vi "MultiPAS-III.vi"() -> ()   [LabVIEW 2011]
uses:
  <vilib>/Analysis/4window.llb/windowTd.ctl
  sub/QMH/QMH Add Message to Queue (Single Element).vi
  sub/QMH/QMH Add Message to Queue (Array).vi
  <vilib>/measure/maspectr.llb/FFT Spectrum (Mag-Phase) for 1 Chan.vi
  sub/fftGetMags.vi
  sub/rollingAverage_III.vi
  sub/micUnbundle_III.vi
  <vilib>/Instr/_visa.llb/VISA Configure Serial Port (Instr).vi
  sub/absCalcPlot_III.vi
  sub/pdNormalize_III.vi
  <vilib>/measure/NI_MAPro.lvlib
  <vilib>/Analysis/NI_AALPro.lvlib
panel:
  out "PAS Save":bool caption="Overtemp"
  in  "Data 2":i32[][](array[numeric])=[[-16374, -7248, 2543, 12030, 20279, 26487, 30037, 30583, 28073, 22744, 15131, 5976, -3818, -13288, -21504, -27663, -31155, -31636, -29064, -23686, -16036, -6862, 2936, 12388, 20571, 26684, 30122, 30546, 27911, 22483, 14793, 5595, -4207, -13644, -21795, -27855, -31232, -31591, -28898, -23423, -15695, -6476, 3323, 12743, 20858, 26873, 30194, 30492, 27744, 22213, 14447, 5207, -4597, -14002, -22082, -28044, -31304, -31540, -28731, -23149, -15348, -6093, 3713, 13101, 21145, 27063, 30265, 30442, 27576, 21943, 14103, 4822, -4984, -14354, -22365, -28230, -31373, -31485, -28556, -22876, -14998, -5702, 4104, 13452, 21428, 27245, 30335, 30388, 27400, 21669, 13754, 4435, -5375, -14705, -22643, -28407, -31436, -31426, -28378, -22598, -14648, -5314, 4497, 13803, 21706, 27423, 30394, 30325, 27221, 21390, 13402, 4045, -5763, -15056, -22921, -28586, -31496, -31361, -28198, -22319, -14297, -4924, 4879, 14151, 21982, 27597, 30451, 30257, 27038, 21107, 13050, 3658, -6149, -15402, -23193, -28754, -31546, -31290, -28010, -22033, -13944, -4536, 5266, 14498, 22252, 27767, 30500, 30184, 26849, 20821, 12696, 3267, -6535, -15748, -23462, -28924, -31596, -31216, -27821, -21748, -13587, -4147, 5653, 14838, 22519, 27930, 30549, 30110, 26658, 20535, 12337, 2878, -6919, -16089, -23727, -29087, -31641, -31137, -27627, -21457, -13229, -3753, 6038, 15181, 22786, 28093, 30591, 30031, 26461, 20243, 11979, 2485, -7303, -16428, -23991, -29244, -31678, -31053, -27426, -21159, -12867, -3360, 6424, 15524, 23043, 28252, 30633, 29946, 26262, 19946, 11617, 2096, -7686, -16764, -24246, -29398, -31712, -30964, -27224, -20862, -12503, -2971, 6803, 15859, 23301, 28401, 30661, 29852, 26058, 19648, 11254, 1703, -8069, -17099, -24500, -29547, -31741, -30870, -27018, -20562, -12138, -2575, 7188, 16192, 23556, 28549, 30689, 29756, 25848, 19348, 10891, 1312, -8448, -17430, -24753, -29691, -31765, -30773, -26806, -20259, -11775, -2186, 7566, 16521, 23801, 28690, 30709, 29656, 25634, 19038, 10523, 919, -8831, -17762, -24997, -29833, -31788, -30672, -26593, -19955, -11409, -1792, 7944, 16850, 24047, 28830, 30724, 29548, 25416, 18729, 10152, 523, -9212, -18092, -25245, -29969, -31805, -30566, -26375, -19647, -11041, -1403, 8319, 17173, 24287, 28963, 30734, 29436, 25192, 18418, 9781, 130, -9587, -18413, -25481, -30101, -31814, -30449, -26150, -19332, -10666, -1007, 8697, 17497, 24524, 29090, 30745, 29325, 24968, 18105, 9408, -263, -9962, -18735, -25718, -30228, -31820, -30334, -25921, -19016, -10296, -618, 9072, 17814, 24756, 29213, 30746, 29202, 24738, 17787, 9036, -657, -10338, -19058, -25951, -30350, -31818, -30214, -25690, -18699, -9922, -224, 9442, 18128, 24984, 29330, 30738, 29078, 24502, 17466, 8658, -1050, -10710, -19371, -26178, -30467, -31814, -30088, -25458, -18382, -9550, 167, 9812, 18440, 25206, 29443, 30732, 28947, 24264, 17143, 8281, -1445, -11083, -19685, -26404, -30581, -31807, -29959, -25221, -18059, -9175, 556, 10178, 18750, 25426, 29548, 30718, 28809, 24018, 16812, 7901, -1842, -11457, -19996, -26624, -30690, -31795, -29824, -24980, -17733, -8799, 950, 10549, 19058, 25643, 29655, 30700, 28673, 23773, 16484, 7523, -2235, -11824, -20304, -26840, -30793, -31772, -29682, -24731, -17402, -8415, 1341, 10916, 19363, 25856, 29755, 30677, 28528, 23522, 16151, 7141, -2626, -12191, -20607, -27051, -30891, -31746, -29536, -24481, -17070, -8035, 1733, 11280, 19664, 26064, 29851, 30648, 28381, 23272, 15818, 6762, -3019, -12555, -20906, -27258, -30984, -31717, -29391, -24226, -16736, -7655, 2128, 11641, 19962, 26270, 29940, 30615, 28229, 23013, 15483, 6376, -3409, -12914, -21204, -27459, -31071, -31684, -29236, -23967, -16398, -7271, 2515, 12005, 20258, 26468, 30024, 30577, 28072, 22753, 15143, 5990, -3802, -13276, -21497, -27660, -31157, -31643, -29076, -23707, -16058, -6886, 2908, 12363, 20550, 26666, 30107, 30536, 27914, 22489, 14805, 5607, -4192, -13633, -21787, -27849, -31230, -31597, -28911, -23438, -15716, -6501, 3298, 12719, 20839, 26858, 30182, 30488, 27744, 22223, 14459, 5225, -4579, -13988, -22071, -28040, -31304, -31549, -28743, -23167, -15368, -6113, 3693, 13076, 21126, 27047, 30255, 30438, 27576, 21950, 14113, 4837, -4971, -14340, -22354, -28224, -31375, -31494, -28570, -22895, -15022, -5725, 4080, 13430, 21408, 27230, 30324, 30384, 27402, 21676, 13766, 4449, -5360, -14694, -22636, -28409, -31440, -31436, -28397, -22617, -14674, -5338, 4467, 13781, 21686, 27408, 30385, 30320, 27224, 21398, 13418, 4062, -5748, -15044, -22913, -28584, -31498, -31368, -28212, -22339, -14321, -4948, 4856, 14131, 21963, 27583, 30440, 30254, 27042, 21118, 13062, 3669, -6137, -15390, -23183, -28751, -31551, -31297, -28024, -22049, -13962, -4556, 5245, 14476, 22235, 27754, 30497, 30186, 26857, 20834, 12710, 3283, -6519, -15733, -23453, -28921, -31600, -31226, -27837, -21765, -13610, -4168, 5628, 14820, 22502, 27918, 30540, 30109, 26664, 20544, 12354, 2891, -6906, -16074, -23719, -29085, -31646, -31148, -27642, -21475, -13251, -3777, 6014, 15160, 22765, 28078, 30583, 30027, 26468, 20251, 11994, 2501, -7292, -16415, -23980, -29242, -31682, -31064, -27443, -21181, -12892, -3386, 6397, 15501, 23026, 28238, 30624, 29944, 26269, 19959, 11633, 2110, -7673, -16753, -24239, -29395, -31719, -30974, -27239, -20882, -12528, -2993, 6782, 15835, 23285, 28390, 30651, 29852, 26063, 19660, 11271, 1720, -8053, -17087, -24493, -29546, -31746, -30880, -27031, -20583, -12163, -2599, 7166, 16173, 23538, 28538, 30684, 29758, 25853, 19356, 10906, 1327, -8433, -17416, -24743, -29688, -31769, -30782, -26821, -20280, -11797, -2208, 7543, 16501, 23786, 28680, 30704, 29656, 25642, 19053, 10540, 936, -8814, -17747, -24989, -29827, -31787, -30678, -26606, -19973, -11430, -1817, 7923, 16829, 24031, 28819, 30721, 29552, 25424, 18746, 10174, 543, -9191, -18072, -25231, -29962, -31802, -30567, -26384, -19660, -11057, -1422, 8302, 17159, 24274, 28952, 30738, 29443, 25205, 18435, 9801, 150, -9568, -18401, -25472, -30095, -31811, -30457, -26163, -19349, -10687, -1031, 8679, 17481, 24511, 29082, 30742, 29327, 24979, 18121, 9431, -241, -9943, -18717, -25707, -30221, -31815, -30337, -25930, -19029, -10312, -631, 9058, 17802, 24745, 29207, 30746, 29209, 24750, 17805, 9057, -634, -10316, -19037, -25937, -30340, -31814, -30217, -25700, -18713, -9939, -240, 9429, 18117, 24976, 29328, 30740, 29088, 24519, 17486, 8682, -1027, -10688, -19352, -26164, -30458, -31810, -30091, -25465, -18390, -9561, 154, 9800, 18433, 25201, 29442, 30735, 28959, 24282, 17165, 8308, -1420, -11063, -19665, -26386, -30570, -31801, -29961, -25227, -18068, -9185, 547, 10171, 18745, 25424, 29552, 30726, 28825, 24038, 16835, 7925, -1815, -11429, -19974, -26608, -30681, -31789, -29826, -24984, -17741, -8807, 938, 10536, 19047, 25636, 29657, 30708, 28685, 23794, 16510, 7550, -2205, -11798, -20280, -26821, -30782, -31766, -29684, -24737, -17411, -8429, 1331, 10906, 19356, 25851, 29758, 30684, 28544, 23546, 16178, 7169, -2598, -12162, -20582, -27035, -30879, -31744, -29540, -24485, -17080, -8048, 1721, 11267, 19655, 26061, 29852, 30654, 28395, 23291, 15843, 6786, -2993, -12527, -20884, -27240, -30974, -31713, -29390, -24230, -16744, -7662, 2115, 11635, 19957, 26268, 29945, 30624, 28246, 23035, 15509, 6406, -3382, -12889, -21180, -27444, -31061, -31677, -29236, -23975, -16408, -7284], [-19329, -1252, 17344, 29341, 30145, 19451, 1353, -17227, -29174, -29920, -19175, -1056, 17506, 29408, 30095, 19300, 1159, -17387, -29238, -29860, -19019, -860, 17671, 29475, 30037, 19143, 960, -17553, -29307, -29809, -18866, -664, 17832, 29545, 29987, 18991, 771, -17707, -29365, -29749, -18707, -466, 17992, 29605, 29926, 18832, 570, -17873, -29434, -29694, -18556, -272, 18151, 29670, 29869, 18676, 375, -18031, -29495, -29633, -18395, -75, 18310, 29729, 29809, 18516, 175, -18194, -29561, -29579, -18238, 120, 18469, 29792, 29750, 18362, -17, -18347, -29617, -29515, -18076, 316, 18629, 29848, 29682, 18197, -218, -18510, -29679, -29456, -17921, 513, 18787, 29910, 29626, 18042, -408, -18664, -29734, -29388, -17757, 709, 18941, 29965, 29560, 17875, -609, -18823, -29791, -29326, -17600, 904, 19095, 30023, 29495, 17717, -802, -18975, -29845, -29260, -17434, 1099, 19251, 30075, 29425, 17551, -1001, -19131, -29901, -29194, -17277, 1296, 19408, 30130, 29359, 17393, -1193, -19284, -29953, -29124, -17112, 1491, 19560, 30184, 29290, 17225, -1392, -19440, -30008, -29056, -16949, 1686, 19713, 30237, 29226, 17069, -1581, -19587, -30054, -28982, -16781, 1883, 19866, 30287, 29151, 16898, -1781, -19742, -30107, -28913, -16616, 2079, 20018, 30337, 29082, 16737, -1973, -19888, -30152, -28838, -16449, 2275, 20167, 30383, 29006, 16564, -2174, -20041, -30200, -28765, -16282, 2471, 20321, 30430, 28934, 16403, -2364, -20187, -30243, -28688, -16113, 2669, 20465, 30470, 28853, 16230, -2568, -20341, -30294, -28618, -15953, 2860, 20615, 30519, 28783, 16070, -2755, -20486, -30335, -28537, -15779, 3057, 20760, 30560, 28700, 15892, -2956, -20637, -30378, -28461, -15613, 3252, 20909, 30605, 28628, 15730, -3145, -20777, -30418, -28377, -15440, 3446, 21054, 30645, 28543, 15557, -3345, -20927, -30460, -28299, -15271, 3643, 21199, 30686, 28465, 15391, -3534, -21066, -30495, -28215, -15100, 3839, 21345, 30722, 28380, 15214, -3734, -21213, -30534, -28134, -14928, 4032, 21487, 30760, 28300, 15044, -3926, -21355, -30570, -28052, -14757, 4225, 21627, 30792, 28209, 14870, -4123, -21501, -30607, -27968, -14586, 4419, 21768, 30832, 28129, 14702, -4314, -21637, -30639, -27880, -14413, 4612, 21907, 30859, 28040, 14521, -4515, -21780, -30675, -27796, -14241, 4804, 22048, 30895, 27953, 14352, -4702, -21919, -30705, -27707, -14064, 4999, 22187, 30922, 27859, 14172, -4900, -22060, -30739, -27620, -13892, 5193, 22326, 30954, 27773, 14003, -5090, -22194, -30765, -27524, -13712, 5386, 22462, 30981, 27679, 13823, -5285, -22333, -30794, -27436, -13538, 5580, 22600, 31013, 27591, 13650, -5476, -22466, -30820, -27343, -13363, 5770, 22732, 31033, 27491, 13468, -5673, -22605, -30848, -27251, -13187, 5964, 22870, 31060, 27401, 13292, -5863, -22736, -30870, -27155, -13010, 6156, 23000, 31079, 27299, 13111, -6058, -22873, -30895, -27060, -12833, 6347, 23134, 31104, 27208, 12936, -6248, -23004, -30918, -26965, -12652, 6536, 23260, 31120, 27106, 12753, -6444, -23136, -30939, -26865, -12472, 6729, 23395, 31148, 27011, 12578, -6634, -23266, -30959, -26766, -12296, 6919, 23523, 31161, 26907, 12392, -6830, -23402, -30982, -26665, -12115, 7109, 23652, 31180, 26809, 12213, -7016, -23524, -30992, -26564, -11932, 7301, 23777, 31195, 26704, 12032, -7210, -23655, -31011, -26464, -11755, 7492, 23907, 31211, 26605, 11855, -7395, -23778, -31024, -26358, -11573, 7680, 24031, 31218, 26494, 11665, -7592, -23908, -31039, -26258, -11392, 7871, 24158, 31237, 26394, 11491, -7775, -24031, -31050, -26153, -11210, 8063, 24281, 31247, 26285, 11302, -7972, -24159, -31062, -26046, -11027, 8250, 24407, 31258, 26180, 11124, -8157, -24276, -31067, -25937, -10841, 8438, 24526, 31265, 26071, 10936, -8347, -24401, -31078, -25829, -10659, 8630, 24649, 31275, 25965, 10755, -8533, -24522, -31087, -25721, -10474, 8816, 24770, 31280, 25853, 10566, -8726, -24641, -31091, -25608, -10290, 9003, 24891, 31287, 25746, 10386, -8910, -24756, -31095, -25498, -10105, 9192, 25008, 31287, 25627, 10196, -9102, -24881, -31101, -25386, -9919, 9381, 25127, 31296, 25521, 10019, -9284, -24994, -31099, -25268, -9732, 9570, 25243, 31293, 25403, 9826, -9476, -25113, -31105, -25157, -9544, 9756, 25359, 31298, 25291, 9645, -9655, -25225, -31099, -25040, -9359, 9942, 25473, 31291, 25167, 9453, -9847, -25341, -31102, -24926, -9173, 10124, 25586, 31294, 25057, 9269, -10029, -25450, -31095, -24809, -8986, 10310, 25696, 31284, 24931, 9078, -10218, -25564, -31094, -24688, -8798, 10497, 25812, 31287, 24819, 8896, -10399, -25673, -31085, -24567, -8608, 10682, 25922, 31278, 24698, 8703, -10587, -25785, -31080, -24448, -8422, 10866, 26033, 31274, 24582, 8522, -10765, -25890, -31067, -24321, -8230, 11050, 26140, 31263, 24455, 8325, -10952, -26001, -31064, -24201, -8040, 11234, 26248, 31255, 24338, 8142, -11132, -26106, -31054, -24079, -7852, 11417, 26353, 31243, 24207, 7948, -11316, -26217, -31041, -23952, -7662, 11601, 26464, 31236, 24089, 7763, -11494, -26315, -31025, -23829, -7471, 11782, 26562, 31217, 23957, 7567, -11682, -26422, -31014, -23702, -7282, 11962, 26667, 31205, 23834, 7383, -11859, -26521, -30998, -23575, -7092, 12144, 26770, 31187, 23704, 7186, -12043, -26626, -30981, -23444, -6900, 12328, 26875, 31176, 23582, 7003, -12218, -26724, -30962, -23316, -6709, 12505, 26971, 31154, 23446, 6805, -12401, -26825, -30946, -23189, -6517, 12687, 27073, 31139, 23322, 6620, -12576, -26919, -30922, -23054, -6323, 12867, 27170, 31114, 23185, 6422, -12760, -27022, -30904, -22923, -6132, 13047, 27272, 31096, 23060, 6237, -12934, -27114, -30879, -22790, -5940, 13222, 27362, 31068, 22921, 6041, -13116, -27212, -30855, -22657, -5748, 13401, 27461, 31048, 22790, 5853, -13289, -27302, -30828, -22522, -5555, 13577, 27549, 31019, 22652, 5652, -13472, -27398, -30806, -22388, -5362, 13753, 27645, 30995, 22521, 5463, -13642, -27487, -30776, -22248, -5169, 13928, 27733, 30963, 22376, 5266, -13823, -27584, -30750, -22113, -4975, 14106, 27828, 30937, 22246, 5082, -13992, -27669, -30717, -21974, -4782, 14280, 27914, 30902, 22101, 4880, -14174, -27760, -30689, -21837, -4588, 14454, 28006, 30875, 21965, 4692, -14340, -27843, -30653, -21693, -4391, 14631, 28092, 30840, 21822, 4494, -14519, -27934, -30620, -21552, -4198, 14805, 28179, 30808, 21688, 4308, -14687, -28015, -30582, -21410, -4004, 14975, 28262, 30770, 21540, 4106, -14861, -28103, -30548, -21268, -3808, 15149, 28349, 30739, 21402, 3916, -15032, -28183, -30512, -21124, -3614, 15319, 28430, 30697, 21255, 3715, -15205, -28267, -30475, -20982, -3421, 15490, 28513, 30664, 21116, 3524, -15376, -28348, -30435, -20837, -3225, 15660, 28592, 30617, 20962, 3327, -15550, -28432, -30397, -20695, -3032, 15829, 28673, 30581, 20820, 3134, -15711, -28506, -30353, -20546, -2837, 15994, 28746, 30530, 20669, 2933, -15887, -28585, -30311, -20400, -2641, 16167, 28828, 30496, 20528, 2745, -16052, -28660, -30264, -20248, -2445, 16335, 28901, 30445, 20376, 2544, -16221, -28737, -30219, -20102, -2250, 16505, 28983, 30406, 20231, 2357, -16381, -28808, -30171, -19950, -2053, 16670, 29053, 30355, 20075, 2154, -16552, -28883, -30127, -19803, -1859, 16835, 29128, 30308, 19930, 1965, -16714, -28952, -30073, -19650, -1663, 17001, 29192, 30255, 19772, 1764, -16881, -29028, -30026, -19496, -1467, 17165, 29268, 30208, 19626, 1572, -17043, -29095, -29977, -19346]]
  out "Filtering":bool caption="Time has Elapsed"
  in  "Switch Filter":bool
  in  "Auto Filter":bool
  out "Elapsed Time (min)":dbl caption="Elapsed Time (s)" format="%#.1g"
  in  "Filter Length (min)":dbl=6.0 caption="Time Target (s)"
  in  "Sample Length (min)":dbl=24.0 caption="Time Target (s)" format="%#.1f"
  out "Time has Elapsed":bool
  in  "Time Target (s)":dbl=1.0
  in  "sweep":bool
  in  "All Emit":bool
  in  "Alignment Mode":bool
  in  "782 Emission":bool
  in  "782 Power (mW)":dbl(slide)=100.0 min=0.0 max=100.0 step=1.0 scale=0.0..100.0
  in  "532 Emission":bool
  in  "532 Power (mW)":dbl(slide)=100.0 min=0.0 max=100.0 step=1.0 scale=0.0..100.0
  in  "423 Power (mW)":dbl(slide)=100.0 min=0.0 max=100.0 step=1.0 scale=0.0..100.0
  in  "423 Emission":bool
  out "Overtemp":bool
  in  "Tab Control":T1(tab)=enum."Frequency Sweep"
  out "Error Console":T2
  out "pd":path caption="Photodiode File Path"
  out "mic":path caption="Microphone File Path"
  out "processed":path caption="Processed Data File Path"
  out "sweeps":path caption="Frequency Sweeps File Path"
  out "Laser Temperatures":T3(graph)
  in  "pd id":u32=1
  in  "mic id":u32
  in  "mic cal, scu":dbl=5.41531278804282e-05 format="%#_3e"
  in  "mic cal, scu":dbl=5.59307241877627e-05 format="%#_3e"
  in  "423 Port":refnum<visa-resource-name>="COM86"
  in  "532 Port":refnum<visa-resource-name>="COM85"
  in  "782 Port":refnum<visa-resource-name>="COM84"
  in  "Teensy Port":refnum<visa-resource-name>="COM87"
  in  "Save Data":bool
  in  "405 PD Cal 3":dbl=0.237
  in  "532 PD Cal 3":dbl=0.454
  in  "660 PD Cal 3":dbl=0.793
  out "freqscan":cluster{i32[], "Best Gaussian Fit":dbl[]}[](graph) caption="Frequency Sweep"
  out "sweep progress":dbl(slide) scale=0.0..1.0
  in  "Autosweep?":bool=TRUE
  in  "set freqs":bool
  out "Calculated Resonance (Hz)":dbl=1370.0
  in  "Data Start Frequency (Hz)":i32=1355
  in  "Data End Frequency (Hz)":i32=1385
  in  "423 F (Hz)":i32=1368
  in  "532 F (Hz)":i32=1372
  in  "785 F (Hz)":i32=1370
  in  "Chart Rolling Average":i32=64
  out "pdwave":waveform(i32)(graph) caption="Photodiode Waveform"
  out "pd ts":cluster{dbl, dbl, dbl}(graph)
  out "pdfft":cluster{"f0":dbl, "df":dbl, "magnitude":dbl[]}(graph) caption="Photodiode FFT"
  in  "rollavg":i32=16 caption="Dispaly Averaging (Transfers to Absorption Data!)"
  out "mic ts":T4(graph)
  out "micfft":cluster{"f0":dbl, "df":dbl, "magnitude":dbl[]}(graph) caption="Photodiode FFT"
  out "micwave":waveform(i32)(graph) caption="Photodiode Waveform"
  in  "getbkg":bool
  out "AAE":dbl(graph)
  in  "Bkg Values (mV)":cluster{dbl, dbl, dbl}
  out "Absorption Spectrum":cluster{dbl[], "Best Power Fit":dbl[]}[](graph)
  out "abs ts":cluster{dbl, dbl, dbl}(graph)
  in  "cellcal":dbl=100000.0 caption="Cell Calibration Coefficient (mV/mW)"
  out "Status":string
  in  "Exit":bool
  in  "State Variables":cluster{"CurrentFile":path}
  # "MultiPAS-IIIir | AeroSmith Labs (2016)"
  # "Laser Control"
  # "Filter Control"
  # "Communications"
  # "Sound Card Parameters"
  # "Data File Options"
  # "File paths are populated automatically at <...\\My Documents\\MultiPAS Data\\>.  To save in another location, turn on \"Save Data\" and follow the prompts to choose an alternate working directory."
  # "Photodiode Calibration"
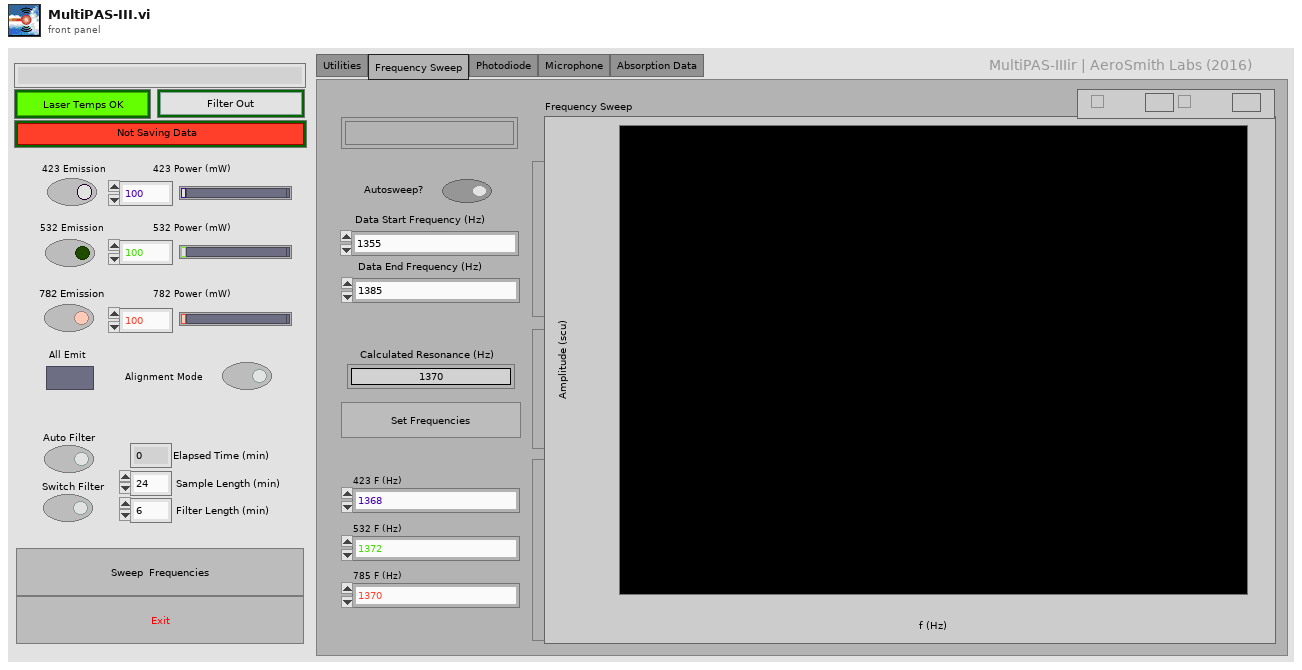
[diagram p1: front panel]
types:
  T1 = enum32{"Utilities", "Frequency Sweep", "Photodiode", "Microphone", "Absorption Data"}
  T2 = cluster{"status":bool, "code":i32, "Message":string}
  T3 = cluster{"Temp (C)":dbl, "Temp (C)":dbl, "Temp (C)":dbl}
  T4 = cluster{"422 Mean":dbl, "532 Mean":dbl, "785 Mean":dbl}
  T5 = cluster{"# buffers":i32, "Buffer size":i32, "unit (ms)":enum16{"time (ms)", "Samples"}}
  T6 = typedef "SoundHandle.ctl" = cluster{"DeviceID":u16, "Samples/buf":u32, "Sampl rate":u32, "Bits/sample":u16, "Channels":u8, "Opened":bool}
  T7 = cluster{"405 Mean":dbl, "532 Mean":dbl, "660 Mean":dbl}
  T8 = typedef "NI_AALPro.lvlib/windowTd.ctl" = u32
  T9 = cluster{"785 New Array":dbl[], "785 Mean":dbl, "785 SD":dbl}
  T10 = cluster{"532 New Array":dbl[], "532 Mean":dbl, "532 SD":dbl}
  T11 = cluster{"422 New Array":dbl[], "422 Mean":dbl, "422 SD":dbl}
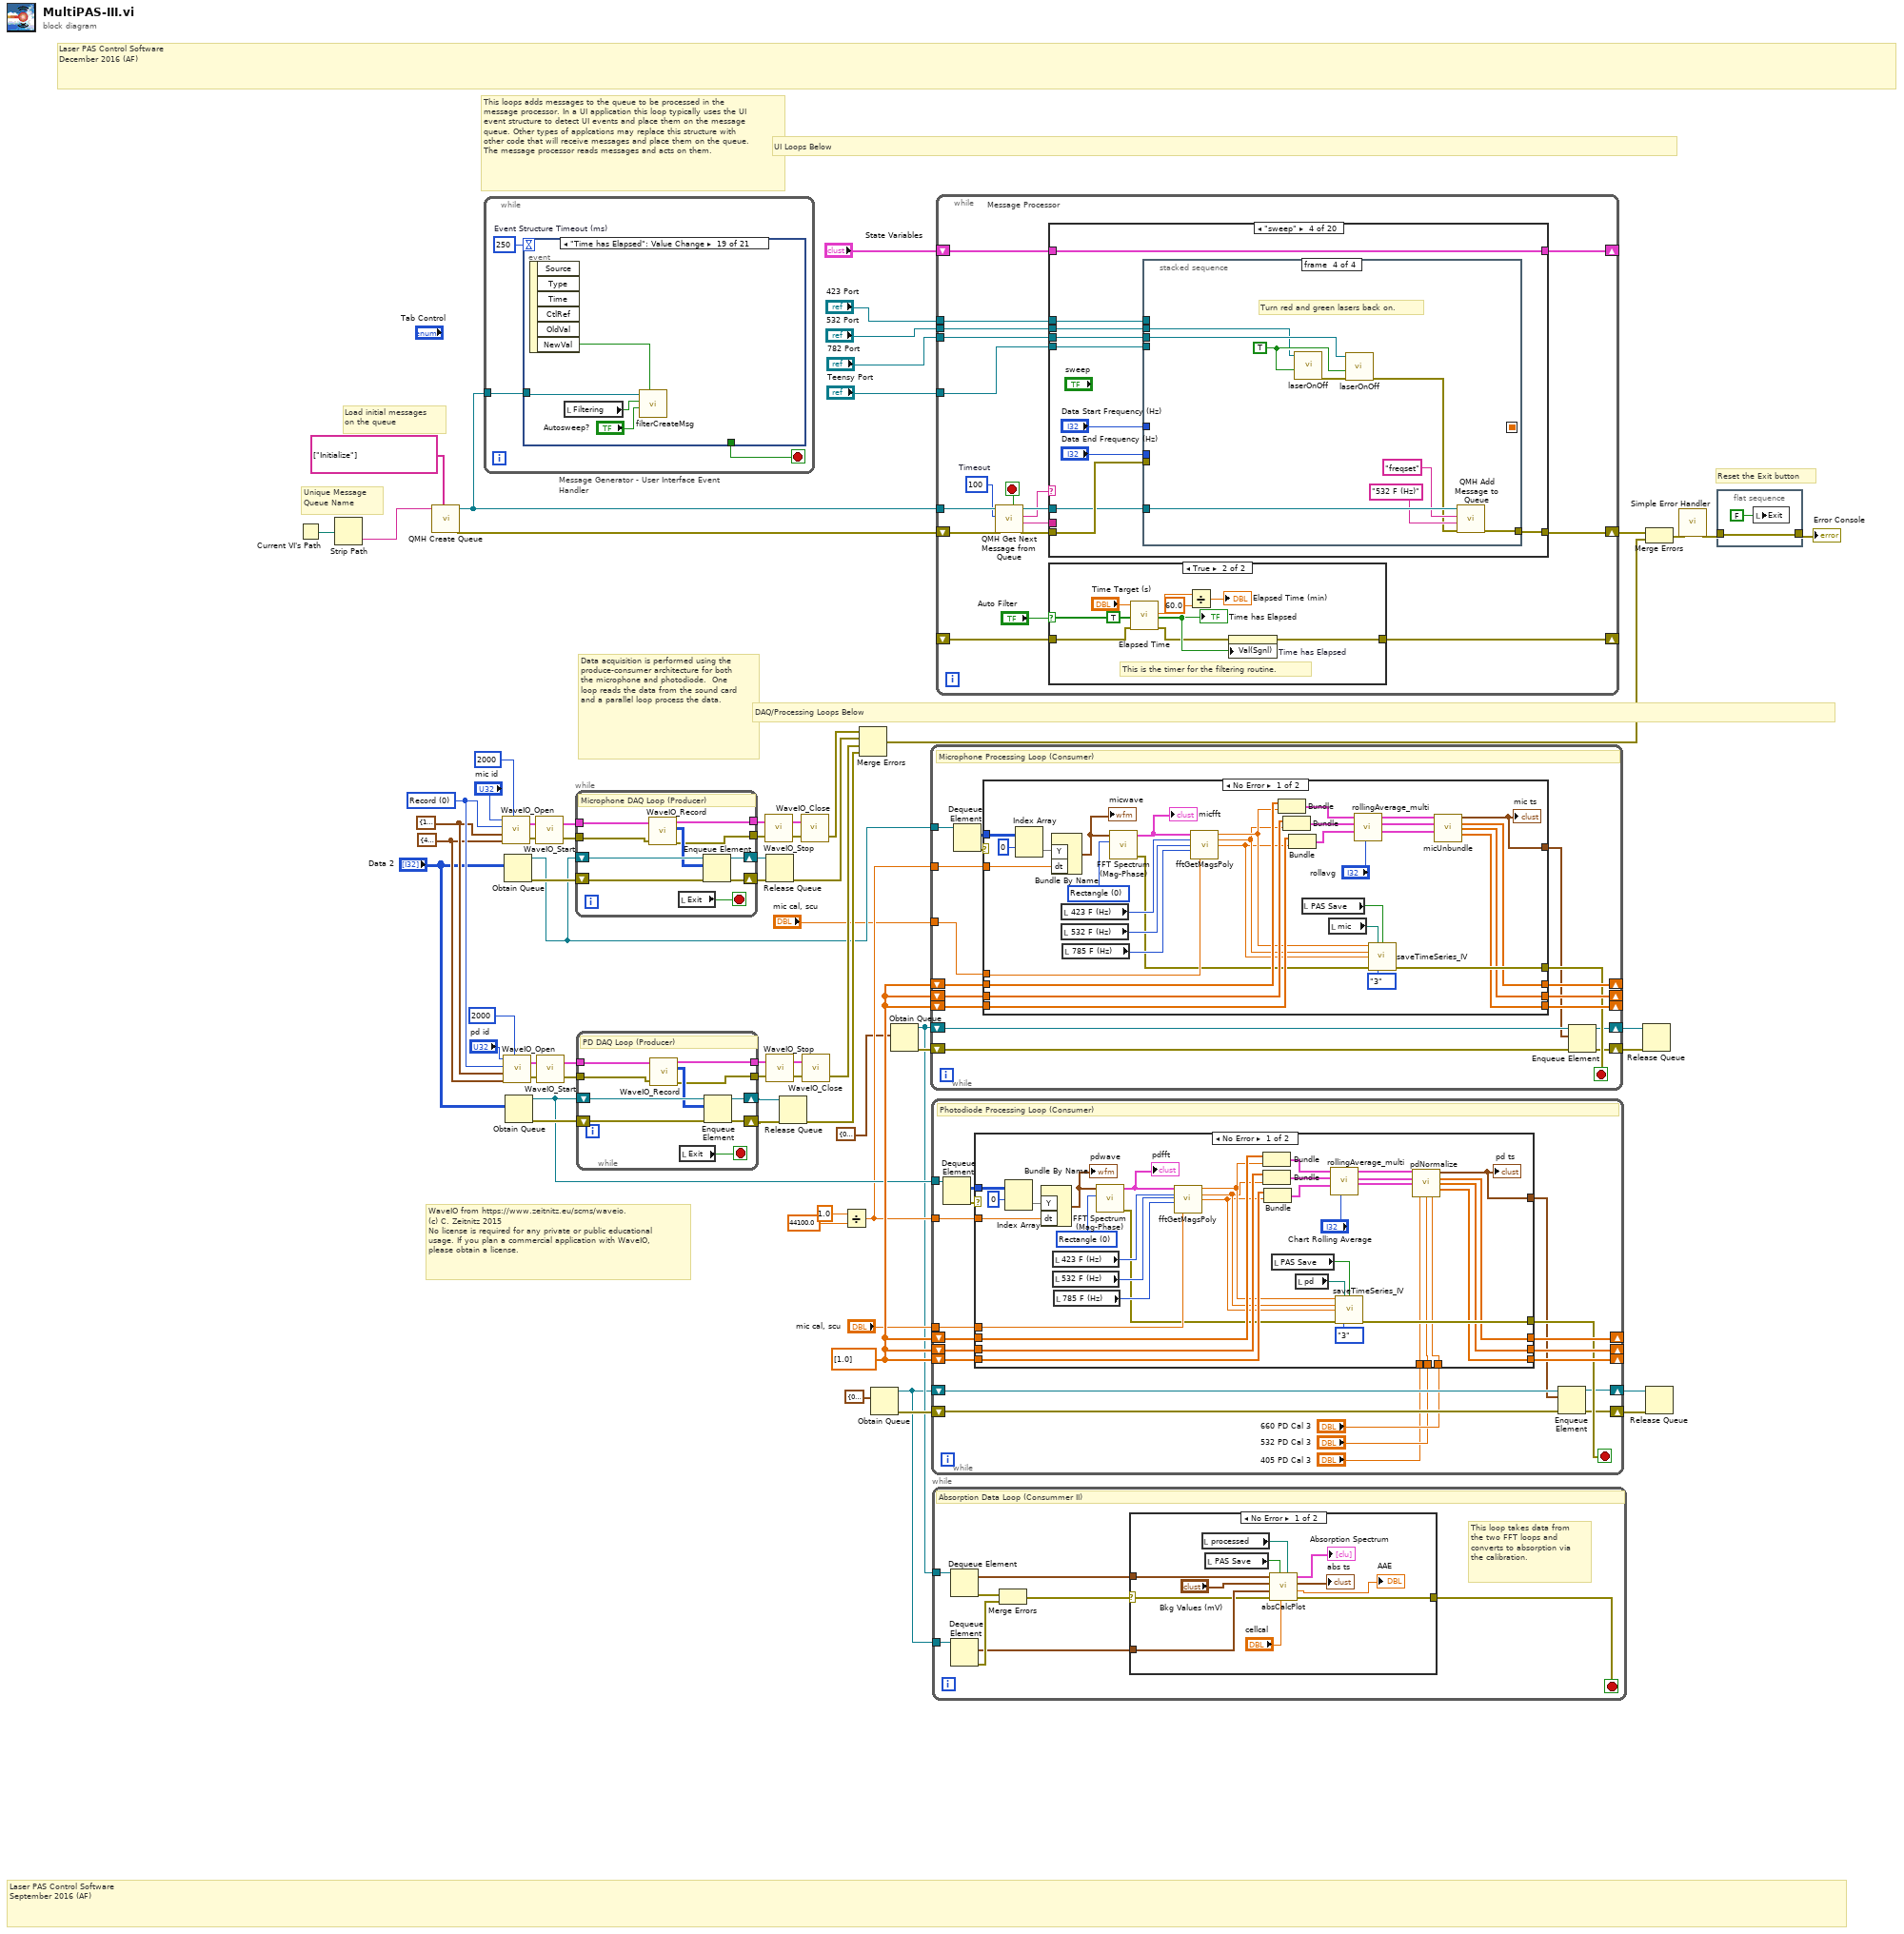
[diagram p0: block diagram]
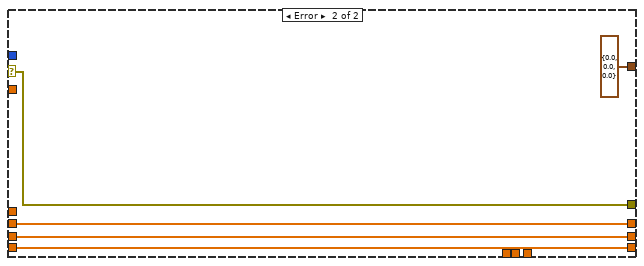
[diagram p3: hidden frame]
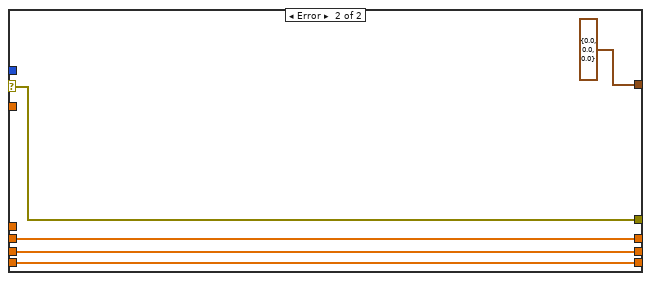
[diagram p4: hidden frame]
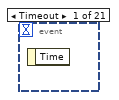
[diagram p5: hidden frame]
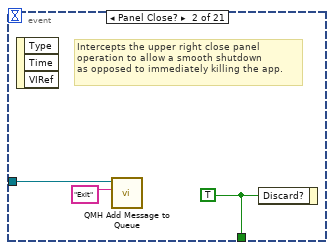
[diagram p6: hidden frame]
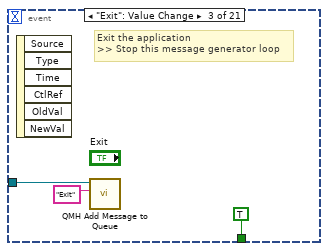
[diagram p7: hidden frame]
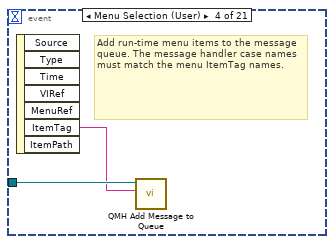
[diagram p8: hidden frame]
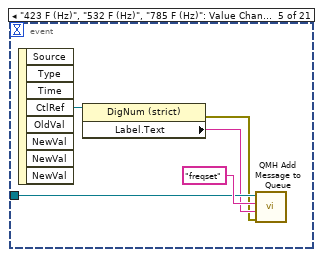
[diagram p9: hidden frame]
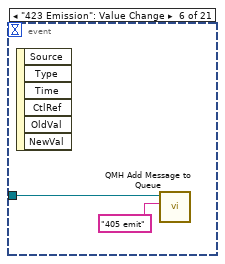
[diagram p10: hidden frame]
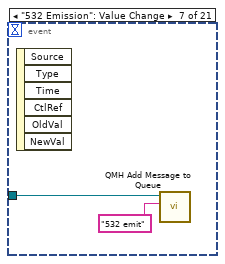
[diagram p11: hidden frame]
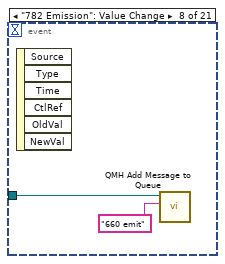
[diagram p12: hidden frame]
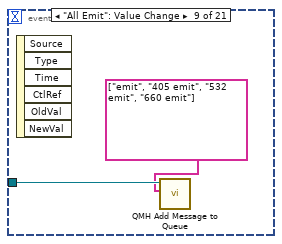
[diagram p13: hidden frame]
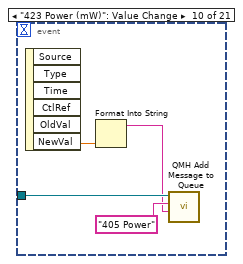
[diagram p14: hidden frame]
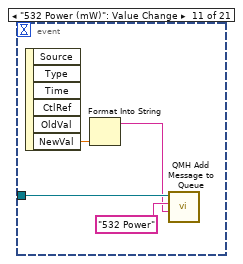
[diagram p15: hidden frame]
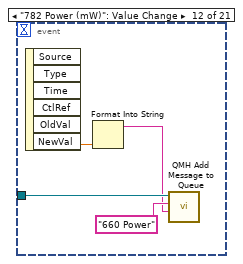
[diagram p16: hidden frame]
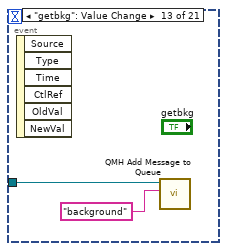
[diagram p17: hidden frame]
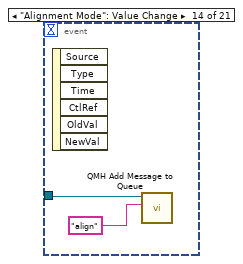
[diagram p18: hidden frame]
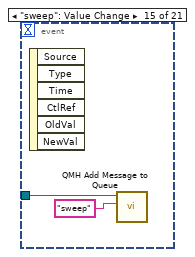
[diagram p19: hidden frame]
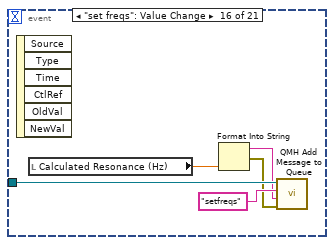
[diagram p20: hidden frame]
diagram:
  w20 = T5 {"# buffers"=10, "Buffer size"=44100, "unit (ms)"=enum."Samples"} ("Buffer")
  w19 = cluster{"Rate":i32, "Bits":i32, "Channels":i32} {"Rate"=44100, "Bits"=24, "Channels"=2} ("Format")
  w21 = u16 0 items=["Record", "Play", "Loopback", "ASIO input", "ASIO output"] ("Direction (Record)")
  w51 = dbl[] [1.0] ("X")
  # "Laser PAS Control Software\nSeptember 2016 (AF)"
  # "Laser PAS Control Software\nDecember 2016 (AF)"
  # "Data acquisition is performed using the produce-consumer architecture for both the microphone and photodiode.  One loop reads the data from the sound card and a parallel loop process the data."
  # "WaveIO from https://www.zeitnitz.eu/scms/waveio.\n(c) C. Zeitnitz 2015\nNo license is required for any private or public educational usage. If you plan a commercial application with WaveIO, please obtain a license."
  # "This loops adds messages to the queue to be processed in the message processor. In a UI application this loop typically uses the UI event structure to detect UI events and place them on the message queue. Other types of applcations may replace this structure with other code that will receive messages and place them on the queue.  The message processor reads messages and acts on them."
  # "Reset the Exit button"
  # "Unique Message\nQueue Name"
  # "Load initial messages\non the queue"
  # "DAQ/Processing Loops Below"
  # "UI Loops Below"
  n1 = Current VI's Path() -> (path=w66:path)
  n2 = Strip Path(path=w66) -> (name=w67:string)  [unwired: 1 out]
  n3 = call "QMH Create Queue.vi"("Initial Messages"=string[] ["Initialize"], "Message queue name (unnamed)"=w67) -> ("error out"=w63:errorcluster, "queue out"=w48:refnum<queue>)  [unwired: 8 in]
  n4 = while "Message Generator - User Interface Event Handler" {
    tunnel: w48 -> [w68]
    stop <- w69 stop-if-true
    w70 = 250  # Event Structure Timeout (ms)
    n5 = event shown="[18] \"Time has Elapsed\": Value Change" {
      selector: _ -> [_ _ _ _ _ _ _ _ _ _ _ _ _ _ _ _ _ _ _ _ _]
      dyn-events: _ -> [_ _ _ _ _ _ _ _ _ _ _ _ _ _ _ _ _ _ _ _ _]
      timeout: w70 -> [_ _ _ _ _ _ _ _ _ _ _ _ _ _ _ _ _ _ _ _ _]
      tunnel: [_ w73 TRUE ("Discard?") _ _ _ _ _ _ _ _ _ _ _ _ _ _ _ _ _ _] -> w69
      tunnel: w68 -> [_ w72 w75 w78 w82 w84 w86 w88 w91 w94 w98 w102 w104 w106 w109 w113 w118 w123 w127 w132 w134]
      event Timeout {
        n6 = event-data() -> ()  [unwired: 1 in, 1 out]
      }
      event Panel Close? {
        w73 = TRUE ("Discard?")
        # "Intercepts the upper right close panel\noperation to allow a smooth shutdown\nas opposed to immediately killing the app."
        n7 = event-data() -> ()  [unwired: 1 in, 3 out]
        n8 = call-poly "QMH Add Message to Queue.vi"("Message"="Exit", "queue in"=w72) -> ()  [unwired: 8 in, 2 out]
        n9 = event-data("Discard?"=w73) -> ()  [unwired: 1 in, 1 out]
      }
      event "Exit": Value Change {
        # "Exit the application\n>> Stop this message generator loop"
        n10 = event-data() -> ()  [unwired: 1 in, 6 out]
        n11 = call-poly "QMH Add Message to Queue.vi"("Message"="Exit", "queue in"=w75) -> ()  [unwired: 8 in, 2 out]
      }
      event Menu Selection (User) {
        # "Add run-time menu items to the message\nqueue. The message handler case names must match the menu ItemTag names."
        n12 = event-data() -> ("ItemTag"=w77:string)  [unwired: 1 in, 6 out]
        n13 = call-poly "QMH Add Message to Queue.vi"("Message"=w77, "queue in"=w78) -> ()  [unwired: 8 in, 2 out]
      }
      event "423 F (Hz)", "532 F (Hz)", "785 F (Hz)": Value Change {
        n14 = event-data() -> ("CtlRef"=w81:refnum<vi>)  [unwired: 1 in, 7 out]
        n15 = property class="DigNum (strict)"(reference=w81) -> (error out=w79:errorcluster, "Label.Text"=w80:string)  [unwired: 1 in, 1 out]
        n16 = call-poly "QMH Add Message to Queue.vi"("error in (no error)"=w79, "Parameter"=w80, "Message"="freqset", "queue in"=w82) -> ()  [unwired: 6 in, 2 out]
      }
      event "423 Emission": Value Change {
        n17 = event-data() -> ()  [unwired: 1 in, 6 out]
        n18 = call-poly "QMH Add Message to Queue.vi"("Message"="405 emit", "queue in"=w84) -> ()  [unwired: 8 in, 2 out]
      }
      event "532 Emission": Value Change {
        n19 = event-data() -> ()  [unwired: 1 in, 6 out]
        n20 = call-poly "QMH Add Message to Queue.vi"("Message"="532 emit", "queue in"=w86) -> ()  [unwired: 8 in, 2 out]
      }
      event "782 Emission": Value Change {
        n21 = event-data() -> ()  [unwired: 1 in, 6 out]
        n22 = call-poly "QMH Add Message to Queue.vi"("Message"="660 emit", "queue in"=w88) -> ()  [unwired: 8 in, 2 out]
      }
      event "All Emit": Value Change {
        n23 = event-data() -> ()  [unwired: 1 in, 6 out]
        n24 = call-poly "QMH Add Message to Queue.vi"("Messages"=string[] ["emit", "405 emit", "532 emit", "660 emit"], "queue in"=w91) -> ()  [unwired: 8 in, 2 out]
      }
      event "423 Power (mW)": Value Change {
        n25 = event-data() -> ("NewVal"=w93:dbl)  [unwired: 1 in, 5 out]
        n26 = Format Into String(w93) -> (resulting string=w92:string)  [unwired: 3 in, 1 out]
        n27 = call-poly "QMH Add Message to Queue.vi"("Parameter"=w92, "Message"="405 Power", "queue in"=w94) -> ()  [unwired: 7 in, 2 out]
      }
      event "532 Power (mW)": Value Change {
        n28 = event-data() -> ("NewVal"=w97:dbl)  [unwired: 1 in, 5 out]
        n29 = Format Into String(w97) -> (resulting string=w96:string)  [unwired: 3 in, 1 out]
        n30 = call-poly "QMH Add Message to Queue.vi"("Parameter"=w96, "Message"="532 Power", "queue in"=w98) -> ()  [unwired: 7 in, 2 out]
      }
      event "782 Power (mW)": Value Change {
        n31 = event-data() -> ("NewVal"=w101:dbl)  [unwired: 1 in, 5 out]
        n32 = Format Into String(w101) -> (resulting string=w100:string)  [unwired: 3 in, 1 out]
        n33 = call-poly "QMH Add Message to Queue.vi"("Parameter"=w100, "Message"="660 Power", "queue in"=w102) -> ()  [unwired: 7 in, 2 out]
      }
      event "getbkg": Value Change {
        n34 = event-data() -> ()  [unwired: 1 in, 6 out]
        n35 = call-poly "QMH Add Message to Queue.vi"("Message"="background", "queue in"=w104) -> ()  [unwired: 8 in, 2 out]
      }
      event "Alignment Mode": Value Change {
        n36 = event-data() -> ()  [unwired: 1 in, 6 out]
        n37 = call-poly "QMH Add Message to Queue.vi"("Message"="align", "queue in"=w106) -> ()  [unwired: 8 in, 2 out]
      }
      event "sweep": Value Change {
        n38 = event-data() -> ()  [unwired: 1 in, 6 out]
        n39 = call-poly "QMH Add Message to Queue.vi"("Message"="sweep", "queue in"=w109) -> ()  [unwired: 8 in, 2 out]
      }
      event "set freqs": Value Change {
        n40 = event-data() -> ()  [unwired: 1 in, 6 out]
        n41 = local read "Calculated Resonance (Hz)"() -> (w112:dbl)
        n42 = Format Into String(w112) -> (resulting string=w111:string, error out=w110:errorcluster)  [unwired: 3 in]
        n43 = call-poly "QMH Add Message to Queue.vi"("error in (no error)"=w110, "Parameter"=w111, "Message"="setfreqs", "queue in"=w113) -> ()  [unwired: 6 in, 2 out]
      }
      event "Save Data": Value Change {
        n44 = event-data() -> ("NewVal"=w117:bool)  [unwired: 1 in, 5 out]
        n45 = Format Into String(w117) -> (resulting string=w116:string, error out=w115:errorcluster)  [unwired: 3 in]
        n46 = call-poly "QMH Add Message to Queue.vi"("error in (no error)"=w115, "Parameter"=w116, "Message"="namefiles", "queue in"=w118) -> ()  [unwired: 6 in, 2 out]
      }
      event "Switch Filter": Value Change {
        n47 = event-data() -> ("NewVal"=w122:bool)  [unwired: 1 in, 5 out]
        n48 = local write "Filtering"(w122) -> ()
        n49 = Format Into String(w122) -> (resulting string=w120:string)  [unwired: 3 in, 1 out]
        n50 = call-poly "QMH Add Message to Queue.vi"("Parameter"=w120, "Message"="filterswitch", "queue in"=w123) -> ()  [unwired: 7 in, 2 out]
      }
      event "Time has Elapsed": Value Change {
        n51 = event-data() -> ("NewVal"=w126:bool)  [unwired: 1 in, 5 out]
        n52 = local read "Filtering"() -> (w125:bool)
        n53 = call "filterCreateMsg.vi"("time elapsed?"=w126, "auto sweep (true)"="Autosweep?", "filtering (true)"=w125, "queue in"=w127) -> ()  [unwired: 6 in, 2 out]
      }
      event "Calculated Resonance (Hz)": Value Change {
        n54 = event-data() -> ("NewVal"=w130:dbl)  [unwired: 1 in, 5 out]
        n55 = Format Into String(w130) -> (resulting string=w128:string, error out=w129:errorcluster)  [unwired: 3 in]
        n56 = call-poly "QMH Add Message to Queue.vi"("error in (no error)"=w129, "Parameter"=w128, "Message"="setfreqs", "queue in"=w132) -> ()  [unwired: 6 in, 2 out]
      }
      event "PAS Save": Value Change {
        n57 = event-data() -> ()  [unwired: 1 in, 6 out]
        n58 = call-poly "QMH Add Message to Queue.vi"("Message"="setwd", "queue in"=w134) -> ()  [unwired: 8 in, 2 out]
      }
    }
  }
  n59 = call <userlib>:"WaveIO_Open.vi"("Watchdog timeout (msec) (default=OFF)"=2000, "Format (44kHz, 16Bit, stereo)"=w19, "Buffer Config"=w20, "Direction (Record)"=w21, "idev"="mic id") -> ("error out"=w44:errorcluster, "Sound Handle Out"=w45:T6)  [unwired: 1 in]
  n60 = call <userlib>:"WaveIO_Open.vi"("Watchdog timeout (msec) (default=OFF)"=2000, "Format (44kHz, 16Bit, stereo)"=w19, "Buffer Config"=w20, "Direction (Record)"=w21, "idev"="pd id") -> ("error out"=w30:errorcluster, "Sound Handle Out"=w29:T6)  [unwired: 1 in]
  n61 = Obtain Queue(element data type="Data 2") -> (queue out=w13:refnum<queue>, error out=w52:errorcluster)  [unwired: 4 in, 1 out]
  n62 = Obtain Queue(element data type="Data 2") -> (queue out=w17:refnum<queue>, error out=w26:errorcluster)  [unwired: 4 in, 1 out]
  n63 = call <userlib>:"WaveIO_Start.vi"("error in (no error)"=w44, "Handle"=w45) -> ("error out"=w42:errorcluster, "Handle Out"=w43:T6)
  n64 = call <userlib>:"WaveIO_Start.vi"("error in (no error)"=w30, "Handle"=w29) -> ("error out"=w32:errorcluster, "Handle Out"=w31:T6)
  n65 = while {
    shift-right: [w143] -> w53
    shift-left: w13 -> [w141]
    shift-right: [w144] -> w54
    shift-left: w52 -> [w142]
    tunnel: w43 -> [w139]
    tunnel: w42 -> [w138]
    tunnel: [w136] -> w39
    tunnel: [w135] -> w38
    stop <- w140 stop-if-true
    # "Microphone DAQ Loop (Producer)"
    n66 = call <userlib>:"WaveIO_Record.vi"("Handle"=w139, "error in (no error)"=w138) -> ("Handle Out"=w136:T6, "Data"=w137:i32[][], "error out"=w135:errorcluster)  [unwired: 1 in, 2 out]
    n67 = local read "Exit"() -> (w140:bool)
    n68 = Enqueue Element(queue=w141, element=w137, error in (no error)=w142) -> (queue out=w143:refnum<queue>, error out=w144:errorcluster)  [unwired: 1 in, 1 out]
  }
  n69 = while {
    shift-right: [w153] -> w25
    shift-left: w17 -> [w151]
    shift-right: [w154] -> w24
    shift-left: w26 -> [w152]
    tunnel: w31 -> [w149]
    tunnel: w32 -> [w148]
    tunnel: [w146] -> w35
    tunnel: [w145] -> w36
    stop <- w150 stop-if-true
    # "PD DAQ Loop (Producer)"
    n70 = call <userlib>:"WaveIO_Record.vi"("Handle"=w149, "error in (no error)"=w148) -> ("Handle Out"=w146:T6, "Data"=w147:i32[][], "error out"=w145:errorcluster)  [unwired: 1 in, 2 out]
    n71 = local read "Exit"() -> (w150:bool)
    n72 = Enqueue Element(queue=w151, element=w147, error in (no error)=w152) -> (queue out=w153:refnum<queue>, error out=w154:errorcluster)  [unwired: 1 in, 1 out]
  }
  n73 = call <userlib>:"WaveIO_Stop.vi"("error in (no error)"=w38, "Handle"=w39) -> ("error out"=w40:errorcluster, "Handle Out"=w41:T6)
  n74 = Release Queue(queue=w53, error in (no error)=w54) -> (error out=w50:errorcluster)  [unwired: 1 in, 2 out]
  n75 = call <userlib>:"WaveIO_Stop.vi"("error in (no error)"=w36, "Handle"=w35) -> ("error out"=w34:errorcluster, "Handle Out"=w33:T6)
  n76 = Release Queue(queue=w25, error in (no error)=w24) -> (error out=w23:errorcluster)  [unwired: 1 in, 2 out]
  n77 = call <userlib>:"WaveIO_Close.vi"("error in (no error)"=w40, "Handle"=w41) -> ("error out"=w37:errorcluster)  [unwired: 1 out]
  n78 = call <userlib>:"WaveIO_Close.vi"("error in (no error)"=w34, "Handle"=w33) -> ("error out"=w22:errorcluster)  [unwired: 1 out]
  n79 = Divide(x=1.0, y=44100.0) -> (x/y=w14:dbl)
  n80 = Merge Errors(w37, w50, w22, w23) -> (w49:errorcluster)
  n81 = Obtain Queue(element data type=cluster{dbl, dbl, dbl} {0.0, 0.0, 0.0}) -> (queue out=w3:refnum<queue>, error out=w7:errorcluster)  [unwired: 4 in, 1 out]
  n82 = Obtain Queue(element data type=cluster{dbl, dbl, dbl} {0.0, 0.0, 0.0}) -> (queue out=w4:refnum<queue>, error out=w10:errorcluster)  [unwired: 4 in, 1 out]
  n83 = while {
    tunnel: w13 -> [w171]
    shift-right: [w168] -> _
    shift-left: w51 -> [w165]
    shift-right: [w167] -> _
    shift-left: w51 -> [w164]
    shift-right: [w166] -> _
    shift-left: w51 -> [w163]
    tunnel: w14 -> [w161]
    tunnel: "mic cal, scu" -> [w160]
    shift-right: [w158] -> w9
    shift-left: w4 -> [w157]
    shift-right: [w155] -> w8
    shift-left: w10 -> [w159]
    stop <- w162 stop-if-true
    # "Microphone Processing Loop (Consumer)"
    n84 = Dequeue Element(queue=w171) -> (element=w169:i32[][], error out=w170:errorcluster)  [unwired: 2 in, 2 out]
    n85 = case shown="No Error" w170 {
      selector: w170 -> [_ w206]
      tunnel: w169 -> [w199 _]
      tunnel: w165 -> [w203 w209]
      tunnel: w164 -> [w202 w207]
      tunnel: w163 -> [w201 w208]
      tunnel: [w175 w209] -> w168
      tunnel: [w174 w207] -> w167
      tunnel: [w173 w208] -> w166
      tunnel: [w182 w206] -> w162
      tunnel: w161 -> [w197 _]
      tunnel: w160 -> [w191 _]
      tunnel: [w176 T7 {"405 Mean"=0.0, "532 Mean"=0.0, "660 Mean"=0.0}] -> w156
      frame No Error {
        w204 = T8 0 items=["Rectangle"=0, "Hanning"=1, "Hamming"=2, "Blackman-Harris"=3, "Exact Blackman"=4, "Blackman"=5, "Flat Top"=6, "4 Term B-Harris "=7, "7 Term B-Harris"=8, "Low Sidelobe"=9, "Blackman Nuttall"=11, "Triangle"=30, "Bartlett-Hanning"=31, "Bohman"=32, "Parzen"=33, "Welch"=34, "Kaiser"=60, "Dolph-Chebyshev"=61, "Gaussian"=62] ("window")
        n86 = Index Array(array=w199, index (row)=0) -> (element=w198:i32[])  [unwired: 1 in]
        n87 = Bundle By Name("Y"=w198, "dt"=w197) -> (w196:waveform(i32))  [unwired: 1 in]
        "micwave" <- w196
        n88 = local read "423 F (Hz)"() -> (w194:i32)
        n89 = local read "532 F (Hz)"() -> (w193:i32)
        n90 = local read "785 F (Hz)"() -> (w192:i32)
        n91 = call-poly <vilib>:"FFT Spectrum (Mag-Phase).vi"("window"=w204, "time signal"=w196) -> ("error out"=w183:errorcluster, "magnitude"=w195:cluster{"f0":dbl, "df":dbl, "magnitude":dbl[]})  [unwired: 5 in, 3 out]
        "micfft" <- w195
        n92 = call-poly "fftGetMagsPoly.vi"("input cluster"=w195, "422 F (Hz)"=w194, "532 F (Hz)"=w193, "785 F (Hz)"=w192, "unit cal, scu"=w191) -> ("mag422 (mV)"=w186:dbl, "mag532 (mV)"=w185:dbl, "mag785 (mV)"=w184:dbl)  [unwired: 8 in]
        n93 = Bundle("X"=w203, "mag422 (mV)"=w186) -> (w190:cluster{"X":dbl[], "mag422 (mV) ":dbl})  [unwired: 1 in]
        n94 = Bundle("X"=w202, "mag532 (mV)"=w185) -> (w189:cluster{"X":dbl[], "mag532 (mV)":dbl})  [unwired: 1 in]
        n95 = Bundle("X"=w201, "mag785 (mV)"=w184) -> (w188:cluster{"X":dbl[], "mag785 (mV)":dbl})  [unwired: 1 in]
        n96 = local read "PAS Save"() -> (w172:bool)
        n97 = local read "mic"() -> (w181:path)
        n98 = call-poly "rollingAverage_multi.vi"("Magnitude Averaging (no. Avgs.)"="rollavg", "785nm"=w188, "532nm"=w189, "422nm"=w190) -> ("785nm Data"=w177:T9, "532nm Data"=w178:T10, "422nm Data"=w179:T11)  [unwired: 5 in]
        n99 = call "saveTimeSeries_IV.vi"("1"=w186, "file path (dialog if empty)"=w181, "save?"=w172, "2"=w185, "3"=w184, "Error In"=w183, "Number of Data Series"=enum16{"1", "2", "3", "4"}."3") -> ("Error Out"=w182:errorcluster)  [unwired: 8 in]
        n100 = call-poly "micUnbundle.vi"("422nm Data"=w179, "532nm Data"=w178, "785nm Data"=w177) -> ("Output Cluster"=w176:T4, "422 New Array"=w175:dbl[], "532 New Array"=w174:dbl[], "785 New Array"=w173:dbl[])  [unwired: 9 in]
        "mic ts" <- w176
      }
      frame Error {
      }
    }
    n101 = Enqueue Element(queue=w157, element=w156, error in (no error)=w159) -> (queue out=w158:refnum<queue>, error out=w155:errorcluster)  [unwired: 1 in, 1 out]
  }
  n102 = while {
    shift-right: [w227] -> _
    shift-left: w51 -> [w224]
    shift-right: [w226] -> _
    shift-left: w51 -> [w223]
    shift-right: [w225] -> _
    shift-left: w51 -> [w222]
    tunnel: w17 -> [w220]
    tunnel: w14 -> [w219]
    tunnel: "mic cal, scu" -> [w218]
    shift-right: [w215] -> w6
    shift-left: w3 -> [w216]
    shift-right: [w214] -> w5
    shift-left: w7 -> [w217]
    stop <- w221 stop-if-true
    # "Photodiode Processing Loop (Consumer)"
    n103 = Dequeue Element(queue=w220) -> (element=w228:i32[][], error out=w229:errorcluster)  [unwired: 2 in, 2 out]
    n104 = case shown="No Error" w229 {
      selector: w229 -> [_ w267]
      tunnel: w228 -> [w260 _]
      tunnel: w224 -> [w264 w270]
      tunnel: w223 -> [w263 w268]
      tunnel: w222 -> [w262 w269]
      tunnel: [w235 w270] -> w227
      tunnel: [w234 w268] -> w226
      tunnel: [w233 w269] -> w225
      tunnel: [w243 w267] -> w221
      tunnel: w219 -> [w258 _]
      tunnel: w218 -> [w252 _]
      tunnel: "660 PD Cal 3" -> [w230 _]
      tunnel: "532 PD Cal 3" -> [w231 _]
      tunnel: "405 PD Cal 3" -> [w232 _]
      tunnel: [w236 cluster{dbl, dbl, dbl} {0.0, 0.0, 0.0}] -> w213
      frame No Error {
        w265 = T8 0 items=["Rectangle"=0, "Hanning"=1, "Hamming"=2, "Blackman-Harris"=3, "Exact Blackman"=4, "Blackman"=5, "Flat Top"=6, "4 Term B-Harris "=7, "7 Term B-Harris"=8, "Low Sidelobe"=9, "Blackman Nuttall"=11, "Triangle"=30, "Bartlett-Hanning"=31, "Bohman"=32, "Parzen"=33, "Welch"=34, "Kaiser"=60, "Dolph-Chebyshev"=61, "Gaussian"=62] ("window")
        n105 = Index Array(array=w260, index (row)=0) -> (element=w259:i32[])  [unwired: 1 in]
        n106 = Bundle By Name("Y"=w259, "dt"=w258) -> (w257:waveform(i32))  [unwired: 1 in]
        "pdwave" <- w257
        n107 = local read "423 F (Hz)"() -> (w255:i32)
        n108 = local read "532 F (Hz)"() -> (w254:i32)
        n109 = local read "785 F (Hz)"() -> (w253:i32)
        n110 = call-poly <vilib>:"FFT Spectrum (Mag-Phase).vi"("window"=w265, "time signal"=w257) -> ("error out"=w244:errorcluster, "magnitude"=w256:cluster{"f0":dbl, "df":dbl, "magnitude":dbl[]})  [unwired: 5 in, 3 out]
        "pdfft" <- w256
        n111 = call-poly "fftGetMagsPoly.vi"("input cluster"=w256, "422 F (Hz)"=w255, "532 F (Hz)"=w254, "785 F (Hz)"=w253, "unit cal, scu"=w252) -> ("mag422 (mV)"=w247:dbl, "mag532 (mV)"=w246:dbl, "mag785 (mV)"=w245:dbl)  [unwired: 8 in]
        n112 = Bundle("X"=w264, "mag422 (mV)"=w247) -> (w251:cluster{"X":dbl[], "mag422 (mV) ":dbl})  [unwired: 1 in]
        n113 = Bundle("X"=w263, "mag532 (mV)"=w246) -> (w250:cluster{"X":dbl[], "mag532 (mV)":dbl})  [unwired: 1 in]
        n114 = Bundle("X"=w262, "mag785 (mV)"=w245) -> (w249:cluster{"X":dbl[], "mag785 (mV)":dbl})  [unwired: 1 in]
        n115 = local read "PAS Save"() -> (w242:bool)
        n116 = local read "pd"() -> (w241:path)
        n117 = call-poly "rollingAverage_multi.vi"("Magnitude Averaging (no. Avgs.)"="Chart Rolling Average", "785nm"=w249, "532nm"=w250, "422nm"=w251) -> ("785nm Data"=w237:T9, "532nm Data"=w238:T10, "422nm Data"=w239:T11)  [unwired: 5 in]
        n118 = call "saveTimeSeries_IV.vi"("1"=w247, "file path (dialog if empty)"=w241, "save?"=w242, "2"=w246, "3"=w245, "Error In"=w244, "Number of Data Series"=enum16{"1", "2", "3", "4"}."3") -> ("Error Out"=w243:errorcluster)  [unwired: 8 in]
        n119 = call-poly "pdNormalize.vi"("422 Data"=w239, "532 Data"=w238, "785 Data"=w237, "422 PD Cal 3"=w232, "532 PD Cal 3"=w231, "785 PD Cal 3"=w230) -> ("pd ts"=w236:cluster{dbl, dbl, dbl}, "422 New Array"=w235:dbl[], "532 New Array"=w234:dbl[], "785 New Array"=w233:dbl[])  [unwired: 6 in]
        "pd ts" <- w236
      }
      frame Error {
      }
    }
    n120 = Enqueue Element(queue=w216, element=w213, error in (no error)=w217) -> (queue out=w215:refnum<queue>, error out=w214:errorcluster)  [unwired: 1 in, 1 out]
  }
  n121 = while {
    tunnel: w4 -> [w272]
    tunnel: w3 -> [w271]
    stop <- w277 stop-if-true
    # "This loop takes data from the two FFT loops and converts to absorption via the calibration."
    # "Absorption Data Loop (Consummer II)"
    n122 = Dequeue Element(queue=w272) -> (element=w278:cluster{dbl, dbl, dbl}, error out=w276:errorcluster)  [unwired: 2 in, 2 out]
    n123 = Dequeue Element(queue=w271) -> (element=w273:cluster{dbl, dbl, dbl}, error out=w275:errorcluster)  [unwired: 2 in, 2 out]
    n124 = Merge Errors(w276, w275) -> (w274:errorcluster)
    n125 = case shown="No Error" w274 {
      selector: w274 -> [w286 w290]
      tunnel: w278 -> [w289 _]
      tunnel: [w285 w290] -> w277
      tunnel: w273 -> [w287 _]
      frame No Error {
        n126 = local read "processed"() -> (w281:path)
        n127 = local read "PAS Save"() -> (w282:bool)
        n128 = call-poly "absCalcPlot.vi"("file path (dialog if empty)"=w281, "Cell Calibration, mV/mW"="cellcal", "save?"=w282, "Error In"=w286, "PD Values"=w287, "bkg values"="Bkg Values (mV)", "Mic Values"=w289) -> ("Error Out"=w285:errorcluster, "aae"=→"AAE":dbl, "Time Series"=→"abs ts":cluster{dbl, dbl, dbl}, "Spectrum"=→"Absorption Spectrum":cluster{dbl[], "Best Power Fit":dbl[]}[])  [unwired: 1 in]
      }
      frame Error {
      }
    }
  }
  n129 = while "Message Processor" {
    shift-left: w63 -> [w303]
    shift-right: [w295] -> w59
    tunnel: w48 -> [w302]
    shift-left: "State Variables" -> [w308]
    shift-right: [w307] -> _
    tunnel: "423 Port" -> [w299]
    tunnel: "532 Port" -> [w298]
    tunnel: "782 Port" -> [w297]
    tunnel: "Teensy Port" -> [w296]
    shift-right: [w293] -> _
    shift-left: _ -> [w292]
    stop <- w306 stop-if-true
    w300 = 100  # Timeout
    n130 = call "QMH Get Next Message from Queue.vi"("error in (no error)"=w303, "ms timeout (1)"=w300, "queue in"=w302) -> ("error out"=w304:errorcluster, "Next Parameter"=w291:string, "Next Message"=w301:string, "queue out"=w305:refnum<queue>, "Stop QMH"=w306:bool)  [unwired: 3 in]
    n131 = case shown="\"sweep\"" w301 {
      selector: w301 -> [_ w335 _ _ _ _ _ _ _ _ _ _ _ _ _ _ _ _ _ _]
      tunnel: [w331 w336 w349 w359 w418 w441 w473 w480 w486 w492 w498 w506 w513 w520 w540 w547 w571 w582 w594 w605] -> w307
      tunnel: w308 -> [w331 w336 w349 w359 w418 w441 w473 w480 w486 w492 w498 w506 w513 w520 w540 w547 w571 w582 w594 w605]
      tunnel: w305 -> [_ _ _ w352 _ _ _ _ _ _ _ _ _ _ _ _ _ _ w592 w606]
      tunnel: w304 -> [w321 w332 w347 w358 w416 w436 w476 w482 w488 w490 w494 w503 w510 w518 w541 w544 w569 w581 w593 w607]
      tunnel: [w320 w332 w338 w351 w415 w438 w472 w478 w484 w490 w497 w504 w511 w514 w541 w543 w568 w581 w590 w596] -> w295
      tunnel: w299 -> [w325 _ w348 w350 _ _ w475 _ _ _ w499 _ _ w517 _ _ _ _ _ w602]
      tunnel: w298 -> [w324 _ w344 w354 _ _ _ w479 _ _ _ w505 _ w516 _ _ _ _ _ w601]
      tunnel: w297 -> [w323 _ w343 w357 _ _ _ _ w485 _ _ _ w512 w515 _ _ _ _ _ w600]
      tunnel: w296 -> [_ _ w341 w353 w417 w439 _ _ _ _ _ _ _ _ _ w545 w570 _ _ w603]
      tunnel: w291 -> [_ _ _ _ w414 w434 _ _ _ _ w496 w500 w507 _ _ _ w567 w580 _ _]
      frame "", "Wait" {
        # "Update the front panel"
        # "Idle Case - this case is called after a Timeout on the Get Next Message from Queue VI, if no new messages are present on the queue. This case can be used for housekeeping tasks such as updating the UI."
        n132 = Get Date/Time String(want seconds? (F)=TRUE) -> (date string=w330:string, time string=w329:string)  [unwired: 2 in]
        n133 = call "laserDiagnose_III.vi"("error in (no error)"=w321, "660 Port 3"=w323, "532 Port in"=w324, "405 Port"=w325) -> ("error out"=w320:errorcluster, "Temperatures"=→"Laser Temperatures":T3, "Overtemp"=→"Overtemp":bool)  [unwired: 3 in, 2 out]
        n134 = Concatenate Strings(w330, " " ("string"), w329) -> (→"Status":string)
      }
      frame Default {
        # "Call this case if a message is received that is not handled \nby any other case. Typically this is a programming error\nas a result of a typo or unhandled message/missing message handler."
        n135 = Format Into String(format string="DevError: Missing message handler for '%s\" message." ("message"), w335) -> (resulting string=w333:string)  [unwired: 2 in, 1 out]
        n136 = One Button Dialog(message=w333) -> ()  [unwired: 1 in, 1 out]
      }
      frame "Initialize" {
        w345 = u32 115200 ("baud rate (9600)")
        # "Initialize the state variables and user interface\nInitialize serial connections"
        n137 = call-poly "VISA Configure Serial Port"("VISA resource name"=w348, "baud rate (9600)"=w345, "error in (no error)"=w347) -> ("error out"=w346:errorcluster)  [unwired: 11 in, 1 out]
        n138 = call-poly "VISA Configure Serial Port"("VISA resource name"=w344, "baud rate (9600)"=w345, "error in (no error)"=w346) -> ("error out"=w342:errorcluster)  [unwired: 11 in, 1 out]
        n139 = call-poly "VISA Configure Serial Port"("VISA resource name"=w343, "baud rate (9600)"=w345, "error in (no error)"=w342) -> ("error out"=w340:errorcluster)  [unwired: 11 in, 1 out]
        n140 = call-poly "VISA Configure Serial Port"("VISA resource name"=w341, "error in (no error)"=w340) -> ("VISA resource name out"=w339:refnum<visa-resource-name>, "error out"=w337:errorcluster)  [unwired: 12 in]
        n141 = property class="Instr" props=["Baud"](reference=w339, error in=w337) -> (error out=w338:errorcluster)  [unwired: 2 out]
      }
      frame "sweep" {
        # "Perform a frequency sweep and calculate the resonance frequency"
        n142 = stacked-sequence {
          seq-local: [_ w372 _ _] -> [_ _ w400 _]
          tunnel: w358 -> [_ w366 _ _]
          tunnel: "Data End Frequency (Hz)" -> [_ w369 w394 _]
          tunnel: "Data Start Frequency (Hz)" -> [_ w368 w393 _]
          tunnel: w357 -> [w362 _ _ w406]
          tunnel: w354 -> [w360 _ _ w405]
          tunnel: w353 -> [_ w367 _ _]
          tunnel: w352 -> [_ _ _ w411]
          tunnel: [_ _ _ w407] -> w351
          tunnel: w350 -> [_ _ _ _]
          frame #0 {
            w365 = FALSE
            # "Turn red and green lasers off for scan."
            n143 = call "laserOnOff.vi"("Emission (F = OFF)"=w365, "VISA Refnum in"=w360) -> ("error out"=w364:errorcluster)  [unwired: 7 in, 2 out]
            n144 = Wait (ms)(milliseconds to wait=u32 5000) -> ()  [unwired: 1 out]
            n145 = local write "Status"("Conducting Frequency Sweep" ("Status")) -> ()
            n146 = call "laserOnOff.vi"("error in (no error)"=w364, "Emission (F = OFF)"=w365, "VISA Refnum in"=w362) -> ()  [unwired: 6 in, 3 out]
          }
          frame #1 {
            n147 = Subtract(x=w369, y=w368) -> (x-y=w370:i32)
            n148 = for {
              N: w370 -> [w376]
              tunnel: [w381] -> w372 mode=indexing
              tunnel: w368 -> [w380]
              tunnel: w369 -> [w379]
              tunnel: w366 -> [_]
              i -> [w373]
              # "Get microphone data."
              # "Listen for N*2000\n seconds"
              n149 = Increment(x=w373) -> (x+1=w374:i32)
              n150 = Divide(x=w374, y=w376) -> (x/y=→"sweep progress":dbl)
              n151 = local read "micfft"() -> (w378:cluster{"f0":dbl, "df":dbl, "magnitude":dbl[]})
              n152 = Unbundle By Name(w378) -> ("magnitude"=w377:dbl[])
              n153 = Wait (ms)(milliseconds to wait=u32 2000) -> ()  [unwired: 1 out]
              n154 = call "fftGetMax.vi"("End Frequency (Hz)"=w379, "Start Frequency (Hz)"=w380, "Magnitudes"=w377) -> ("max value"=w381:dbl)  [unwired: 8 in]
            }
            n155 = case shown="False" TRUE ("sweep?") {
              tunnel: w368 -> [_ w388]
              tunnel: w369 -> [_ w387]
              tunnel: w367 -> [_ w386]
              tunnel: [w383 w385] -> _
              tunnel: w366 -> [w383 w384]
              frame False {
              }
              frame True {
                # "Scan laser freq.\nwith Teensy"
                n156 = call "teensySweepFreq.vi"("error in (no error)"=w384, "end f, Hz (1385)"=w387, "start f, Hz (1355)"=w388, "VISA Refnum in"=w386) -> ("error out"=w385:errorcluster)  [unwired: 7 in]
              }
            }
          }
          frame #2 {
            # "Calculate resonance frequency;\ndisplay and save scan."
            n157 = Wait (ms)(milliseconds to wait=u32 5000) -> ()  [unwired: 1 out]
            n158 = local read "PAS Save"() -> (w389:bool)
            n159 = To Double Precision Float(number=w394) -> (double precision float=w391:dbl)
            n160 = To Double Precision Float(number=w393) -> (double precision float=w392:dbl)
            n161 = call "resCalc.vi"("Frequency Sweep"=w400, "Start F, Hz (1355)"=w393) -> ("F-res, Hz"=w398:dbl, "Frequency Scan"=w390:cluster{i32[], "Best Gaussian Fit":dbl[]}[])  [unwired: 8 in]
            "freqscan" <- w390
            n162 = In Range and Coerce(upper limit=w391, x=w398, lower limit=w392) -> (In Range?=w397:bool)  [unwired: 1 out]
            n163 = case shown="True" w389 {
              tunnel: w390 -> [_ w404]
              tunnel: w398 -> [_ w403]
              frame False {
              }
              frame True {
                n164 = local read "sweeps"() -> (w402:path)
                n165 = call "saveFreqSweep.vi"("f-res, Hz"=w403, "Frequency Scan"=w404, "file path (dialog if empty)"=w402) -> ()  [unwired: 9 in]
              }
            }
            n166 = And(x=w397, y=TRUE ("check freqs?")) -> (x .and. y?=w395:bool)
            n167 = case shown="True" w395 {
              tunnel: w398 -> [_ w401]
              frame False {
              }
              frame True {
                n168 = property on="Calculated Resonance (Hz)" class="DigNum (strict)"("Val(Sgnl)"=w401) -> ()  [unwired: 2 in, 2 out]
                "Calculated Resonance (Hz)" <- w401
              }
            }
          }
          frame #3 {
            w412 = TRUE
            # "Turn red and green lasers back on."
            n169 = call "laserOnOff.vi"("Emission (F = OFF)"=w412, "VISA Refnum in"=w405) -> ("error out"=w413:errorcluster)  [unwired: 7 in, 2 out]
            n170 = call "laserOnOff.vi"("error in (no error)"=w413, "Emission (F = OFF)"=w412, "VISA Refnum in"=w406) -> ("error out"=w408:errorcluster)  [unwired: 6 in, 2 out]
            n171 = call-poly "QMH Add Message to Queue.vi"("error in (no error)"=w408, "Parameter"="532 F (Hz)", "Message"="freqset", "queue in"=w411) -> ("error out"=w407:errorcluster)  [unwired: 6 in, 1 out]
          }
        }
      }
      frame "freqset" {
        # "Set the frequency of the Teensy's modulation\nsignal for single laser (if single frequency is changed)."
        # "Set the laser frequency.  Case for \"red\", \"blue\", or \"green\"."
        n172 = case shown="\"532 F (Hz)\"" w414 {
          tunnel: w416 -> [w423 w428 w432]
          tunnel: [w422 w427 w431] -> w415
          tunnel: w417 -> [w419 w424 w429]
          frame "405 F (Hz) ", Default {
            w421 = u16 0 items=["blue", "green", "red"] ("laser")
            n173 = call "freqSet.vi"("error in (no error)"=w423, "laser"=w421, "Freq, Hz (1370)"="423 F (Hz)", "Teensy Port"=w419) -> ("error out"=w422:errorcluster)  [unwired: 6 in, 1 out]
          }
          frame "532 F (Hz)" {
            w426 = u16 1 items=["blue", "green", "red"] ("laser")
            n174 = call "freqSet.vi"("error in (no error)"=w428, "laser"=w426, "Freq, Hz (1370)"="532 F (Hz)", "Teensy Port"=w424) -> ("error out"=w427:errorcluster)  [unwired: 6 in, 1 out]
          }
          frame "660 F (Hz)" {
            w433 = u16 2 items=["blue", "green", "red"] ("laser")
            n175 = call "freqSet.vi"("error in (no error)"=w432, "laser"=w433, "Freq, Hz (1370)"="785 F (Hz)", "Teensy Port"=w429) -> ("error out"=w431:errorcluster)  [unwired: 6 in, 1 out]
          }
        }
      }
      frame "setfreqs" {
        # "Set the frequency of the Teensy's modulation\nsignal for all lasers at once."
        # "Set laser frequencies to resonance frequency calculated in sweep."
        n176 = Scan From String(input string=w434, error in=w436) -> (error out=w435:errorcluster, output 1=w437:dbl)  [unwired: 3 in, 2 out]
        n177 = for {
          N: 3 -> [_]
          tunnel: [w447] -> w438
          tunnel: w435 -> [w446]
          tunnel: w439 -> [w443]
          tunnel: w437 -> [w445]
          i -> [w444]
          n178 = flat-sequence {
            tunnel: w443 -> [w448]
            tunnel: [w448] -> w442
            frame #0 {
              n179 = Wait (ms)(milliseconds to wait=u32 1000) -> ()  [unwired: 1 out]
            }
          }
          n180 = case shown="1, Default" w444 {
            tunnel: [w455 w463 w471] -> w447
            tunnel: w446 -> [w453 w460 w468]
            tunnel: w442 -> [w452 w459 w467]
            tunnel: w445 -> [w450 w456 w464]
            frame 0 {
              w454 = u16 2 items=["blue", "green", "red"] ("laser")
              n181 = To Long Integer(number=w450) -> (32bit integer=w451:i32)
              n182 = local write "785 F (Hz)"(w451) -> ()
              n183 = call "freqSet.vi"("error in (no error)"=w453, "laser"=w454, "Freq, Hz (1370)"=w451, "Teensy Port"=w452) -> ("error out"=w455:errorcluster)  [unwired: 6 in, 1 out]
            }
            frame 1, Default {
              w462 = u16 1 items=["blue", "green", "red"] ("laser")
              n184 = Add(x=w456, y=2.0) -> (x+y=w458:dbl)
              n185 = To Long Integer(number=w458) -> (32bit integer=w457:i32)
              n186 = call "freqSet.vi"("error in (no error)"=w460, "laser"=w462, "Freq, Hz (1370)"=w457, "Teensy Port"=w459) -> ("error out"=w463:errorcluster)  [unwired: 6 in, 1 out]
              n187 = local write "532 F (Hz)"(w457) -> ()
            }
            frame 2 {
              w470 = u16 0 items=["blue", "green", "red"] ("laser")
              n188 = Subtract(x=w464, y=2.0) -> (x-y=w466:dbl)
              n189 = To Long Integer(number=w466) -> (32bit integer=w465:i32)
              n190 = call "freqSet.vi"("error in (no error)"=w468, "laser"=w470, "Freq, Hz (1370)"=w465, "Teensy Port"=w467) -> ("error out"=w471:errorcluster)  [unwired: 6 in, 1 out]
              n191 = local write "423 F (Hz)"(w465) -> ()
            }
          }
        }
      }
      frame "405 emit" {
        # "Turn laser on or off"
        n192 = call "laserOnOff.vi"("error in (no error)"=w476, "Emission (F = OFF)"="423 Emission", "Power, mW (100)"="423 Power (mW)", "VISA Refnum in"=w475) -> ("error out"=w472:errorcluster)  [unwired: 5 in, 2 out]
      }
      frame "532 emit" {
        # "Turn laser on or off"
        n193 = call "laserOnOff.vi"("error in (no error)"=w482, "Emission (F = OFF)"="532 Emission", "Power, mW (100)"="532 Power (mW)", "VISA Refnum in"=w479) -> ("error out"=w478:errorcluster)  [unwired: 5 in, 2 out]
      }
      frame "660 emit" {
        # "Turn laser on or off"
        n194 = call "laserOnOff.vi"("error in (no error)"=w488, "Emission (F = OFF)"="782 Emission", "Power, mW (100)"="782 Power (mW)", "VISA Refnum in"=w485) -> ("error out"=w484:errorcluster)  [unwired: 5 in, 2 out]
      }
      frame "emit" {
        # "Turn on all lasers."
        n195 = local write "423 Emission"("All Emit") -> ()
        n196 = local write "532 Emission"("All Emit") -> ()
        n197 = local write "782 Emission"("All Emit") -> ()
      }
      frame "405 Power" {
        # "Set laser power"
        n198 = Scan From String(input string=w496, error in=w494) -> (error out=w493:errorcluster, output 1=w495:dbl)  [unwired: 3 in, 2 out]
        n199 = call "laserSetPower.vi"("error in (no error)"=w493, "Laser Power (mW)"=w495, "VISA Refnum in"=w499) -> ("error out"=w497:errorcluster)  [unwired: 7 in, 1 out]
      }
      frame "532 Power" {
        n200 = Scan From String(input string=w500, error in=w503) -> (error out=w502:errorcluster, output 1=w501:dbl)  [unwired: 3 in, 2 out]
        n201 = call "laserSetPower.vi"("error in (no error)"=w502, "Laser Power (mW)"=w501, "VISA Refnum in"=w505) -> ("error out"=w504:errorcluster)  [unwired: 7 in, 1 out]
      }
      frame "660 Power" {
        n202 = Scan From String(input string=w507, error in=w510) -> (error out=w509:errorcluster, output 1=w508:dbl)  [unwired: 3 in, 2 out]
        n203 = call "laserSetPower.vi"("error in (no error)"=w509, "Laser Power (mW)"=w508, "VISA Refnum in"=w512) -> ("error out"=w511:errorcluster)  [unwired: 7 in, 1 out]
      }
      frame "align" {
        # "Set power of all lasers to 5 mW for alignment"
        n204 = case shown="True" "Alignment Mode" {
          tunnel: w518 -> [w528 w538]
          tunnel: w517 -> [w527 w537]
          tunnel: w516 -> [w526 w536]
          tunnel: w515 -> [w525 w535]
          tunnel: [w522 w532] -> w514
          frame True {
            w521 = 5.0 ("Laser Power (mW)")
            n205 = call "laserSetPower.vi"("error in (no error)"=w528, "Laser Power (mW)"=w521, "VISA Refnum in"=w527) -> ("error out"=w524:errorcluster)  [unwired: 7 in, 1 out]
            n206 = call "laserSetPower.vi"("error in (no error)"=w524, "Laser Power (mW)"=w521, "VISA Refnum in"=w526) -> ("error out"=w523:errorcluster)  [unwired: 7 in, 1 out]
            n207 = call "laserSetPower.vi"("error in (no error)"=w523, "Laser Power (mW)"=w521, "VISA Refnum in"=w525) -> ("error out"=w522:errorcluster)  [unwired: 7 in, 1 out]
          }
          frame False, Default {
            n208 = local read "423 Power (mW)"() -> (w531:dbl)
            n209 = local read "532 Power (mW)"() -> (w530:dbl)
            n210 = local read "782 Power (mW)"() -> (w529:dbl)
            n211 = call "laserSetPower.vi"("error in (no error)"=w538, "Laser Power (mW)"=w531, "VISA Refnum in"=w537) -> ("error out"=w534:errorcluster)  [unwired: 7 in, 1 out]
            n212 = call "laserSetPower.vi"("error in (no error)"=w534, "Laser Power (mW)"=w530, "VISA Refnum in"=w536) -> ("error out"=w533:errorcluster)  [unwired: 7 in, 1 out]
            n213 = call "laserSetPower.vi"("error in (no error)"=w533, "Laser Power (mW)"=w529, "VISA Refnum in"=w535) -> ("error out"=w532:errorcluster)  [unwired: 7 in, 1 out]
          }
        }
      }
      frame "background" {
        n214 = local read "mic ts"() -> (w539:T4)
        n215 = local write "Bkg Values (mV)"(w539) -> ()
      }
      frame "filter" {
        n216 = local read "Filtering"() -> (w546:bool)
        n217 = case shown="True" w546 {
          tunnel: w545 -> [w550 w559]
          tunnel: w544 -> [w549 w557]
          tunnel: [w548 w558] -> w543
          frame False {
            n218 = Multiply(x="Filter Length (min)", y=60.0) -> (x*y=w553:dbl)
            n219 = local write "Time Target (s)"(w553) -> ()
            n220 = VISA Write(VISA resource name=w550, write buffer="v.1", error in (no error)=w549) -> (error out=w548:errorcluster)  [unwired: 2 out]
            "Filtering" <- TRUE
          }
          frame True {
            n221 = flat-sequence {
              tunnel: w557 -> [w565]
              tunnel: [w565] -> w556
              frame #0 {
                n222 = local read "mic ts"() -> (w566:T4)
                n223 = local write "Bkg Values (mV)"(w566) -> ()
              }
            }
            n224 = local write "Filtering"(FALSE) -> ()
            n225 = VISA Write(VISA resource name=w559, write buffer="v.0", error in (no error)=w556) -> (error out=w558:errorcluster)  [unwired: 2 out]
            n226 = Multiply(x="Sample Length (min)", y=60.0) -> (x*y=w561:dbl)
            n227 = local write "Time Target (s)"(w561) -> ()
          }
        }
        n228 = Wait (ms)(milliseconds to wait=u32 500) -> ()  [unwired: 1 out]
      }
      frame "filterswitch" {
        n229 = case shown="\"TRUE\"" w567 {
          tunnel: w570 -> [w574 w579]
          tunnel: w569 -> [w573 w578]
          tunnel: [w572 w577] -> w568
          frame "FALSE", Default {
            n230 = VISA Write(VISA resource name=w574, write buffer="v.0", error in (no error)=w573) -> (error out=w572:errorcluster)  [unwired: 2 out]
          }
          frame "TRUE" {
            n231 = VISA Write(VISA resource name=w579, write buffer="v.1", error in (no error)=w578) -> (error out=w577:errorcluster)  [unwired: 2 out]
          }
        }
      }
      frame "namefiles" {
        n232 = case shown="\"TRUE\"" w580 {
          frame "FALSE", Default {
            n233 = local write "PAS Save"(FALSE ("PAS Save")) -> ()
          }
          frame "TRUE" {
            n234 = flat-sequence {
              frame #0 {
                n235 = call "saveSetDirectory.vi"() -> ("mic"=→"mic":path, "pd"=→"pd":path, "processed"=→"processed":path, "sweeps"=→"sweeps":path)  [unwired: 11 in, 1 out]
              }
              frame #1 {
                "PAS Save" <- TRUE ("PAS Save")
              }
            }
          }
        }
      }
      frame "Error" {
        (unwired) errorcluster {"status"=FALSE, "code"=0, "source"=""} ("error out")
        # "Proceed to Exit - remove if this is\nnot appropriate for the General Error case"
        # "General Error Case - this case is called if an error is passed using the error cluster below. Typically most new errors should be handed in each individual case and not passed in the rror cluster. If necessary a custom error handler case should be added and called from other cases."
        n236 = call <vilib>:"Simple Error Handler.vi"("error in (no error)"=w593) -> ("error out"=w589:errorcluster)  [unwired: 4 in, 4 out]
        n237 = call-poly "QMH Add Message to Queue.vi"("error in (no error)"=w589, "Message"="Exit", "queue in"=w592) -> ("error out"=w590:errorcluster)  [unwired: 7 in, 1 out]
      }
      frame "Exit" {
        # "Perform cleanup tasks: Close serial connections and clear front panel."
        n238 = call "QMH Destroy Queue.vi"("error in (no error)"=w607, "queue in"=w606) -> ("error out"=w599:errorcluster)  [unwired: 7 in, 2 out]
        n239 = for {
          N: 3 -> [_]
          tunnel: w602 -> [w614]
          tunnel: w601 -> [w612]
          tunnel: w600 -> [w611]
          tunnel: w599 -> [w610]
          tunnel: FALSE -> [w609]
          tunnel: [w608] -> w595
          i -> [w613]
          # "Close laser serial connections."
          n240 = case shown="0, Default" w613 {
            tunnel: [w621 w626 w631] -> w616
            tunnel: [w620 w625 w630] -> w615
            tunnel: w614 -> [w619 _ _]
            tunnel: w612 -> [_ w624 _]
            tunnel: w611 -> [_ _ w628]
            tunnel: w610 -> [w618 w623 w629]
            tunnel: w609 -> [w617 w622 w627]
            frame 0, Default {
              n241 = call "laserOnOff.vi"("error in (no error)"=w618, "Emission (F = OFF)"=w617, "VISA Refnum in"=w619) -> ("error out"=w621:errorcluster, "VISA Refnum out"=w620:refnum<visa-resource-name>)  [unwired: 6 in, 1 out]
              n242 = local write "423 Emission"(w617) -> ()
            }
            frame 1 {
              n243 = call "laserOnOff.vi"("error in (no error)"=w623, "Emission (F = OFF)"=w622, "VISA Refnum in"=w624) -> ("error out"=w626:errorcluster, "VISA Refnum out"=w625:refnum<visa-resource-name>)  [unwired: 6 in, 1 out]
              n244 = local write "532 Emission"(w622) -> ()
            }
            frame 2 {
              n245 = call "laserOnOff.vi"("error in (no error)"=w629, "Emission (F = OFF)"=w627, "VISA Refnum in"=w628) -> ("error out"=w631:errorcluster, "VISA Refnum out"=w630:refnum<visa-resource-name>)  [unwired: 6 in, 1 out]
              n246 = local write "782 Emission"(w627) -> ()
              n247 = local write "All Emit"(w627) -> ()
            }
          }
          n248 = VISA Close(VISA resource name=w615, error in (no error)=w616) -> (error out=w608:errorcluster)
        }
        n249 = local write "Status"("" ("Status")) -> ()
        n250 = VISA Close(VISA resource name=w603, error in (no error)=w595) -> (error out=w596:errorcluster)
      }
    }
    n251 = case shown="True" "Auto Filter" {
      tunnel: [w309 w311] -> w293
      tunnel: w292 -> [w309 w310]
      frame False {
      }
      frame True {
        # "This is the timer for the filtering routine."
        n252 = call "Elapsed Time"("Time Target (s)"="Time Target (s)", "Auto Reset"=TRUE, "error in (no error)"=w310) -> ("Elapsed Time (s)"=w314:dbl, "Time has Elapsed"=w316:bool, "error out"=w315:errorcluster)  [unwired: 9 in, 5 out]
        "Time has Elapsed" <- w316
        n253 = Divide(x=w314, y=60.0) -> (x/y=→"Elapsed Time (min)":dbl)
        n254 = property on="Time has Elapsed" class="Bool (strict)"(error in=w315, "Val(Sgnl)"=w316) -> (error out=w311:errorcluster)  [unwired: 1 in, 1 out]
      }
    }
  }
  n255 = Release Queue(queue=w9, error in (no error)=w8) -> ()  [unwired: 1 in, 3 out]
  n256 = Merge Errors(w59, w49) -> (w58:errorcluster)
  n257 = Release Queue(queue=w6, error in (no error)=w5) -> ()  [unwired: 1 in, 3 out]
  n258 = call <vilib>:"Simple Error Handler.vi"("error in (no error)"=w58) -> ("error out"=w57:errorcluster)  [unwired: 4 in, 4 out]
  n259 = flat-sequence {
    tunnel: w57 -> [w632]
    tunnel: [w632] -> w56
    frame #0 {
      n260 = local write "Exit"(FALSE) -> ()
    }
  }
  "Error Console" <- w56
